vi "Test Animal Cannot Eat after Eating.vi"(8 "error in (no error)":errorcluster, 11 "Animal Test In":refnum<class "Animal Test.lvclass">) -> (0 "error out":errorcluster, 3 "Animal Test Out":refnum<class "Animal Test.lvclass">)   [LabVIEW 2020, in "Animal Test.lvclass"]
doc: "Test Animal cannot eat after eating."
uses:
  Animal Test.lvclass
  C:/Program Files (x86)/National Instruments/LabVIEW 2020/vi.lib/Astemes/LUnit/Test Case.lvclass
  Animal Test.lvclass/Animal Test.ctl
  <vilib>/Astemes/LUnit/Test Case.lvclass/Test Case.ctl
  092653db-4d85-4f60-a039-c6abd7f22ebd.vi
  <vilib>/Astemes/LUnit/Append Fail Result.vi
  <vilib>/Astemes/LUnit/Append Pass Result.vi
  <vilib>/Astemes/LUnit/Compare Variants.vi
  <vilib>/Astemes/LUnit/Describe Comparison.vi
  <vilib>/Astemes/LUnit/Run In UI.vi
  <vilib>/Utility/error.llb/Clear Errors.vi
  <vilib>/Astemes/LUnit/Describe Variant.vi
  Animal Classes/Animal/Animal.lvclass
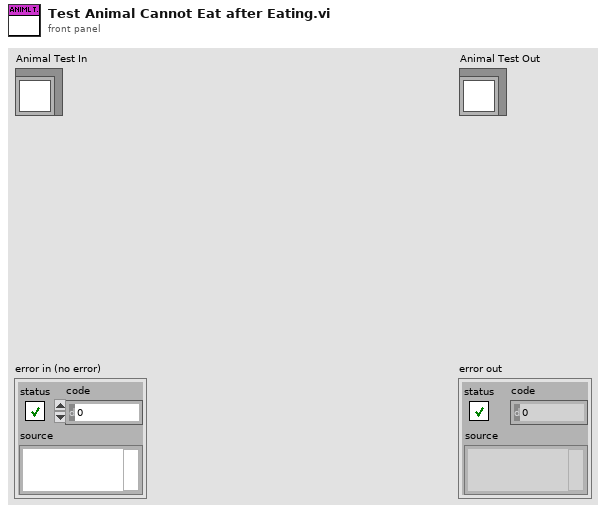
[diagram p1: front panel]
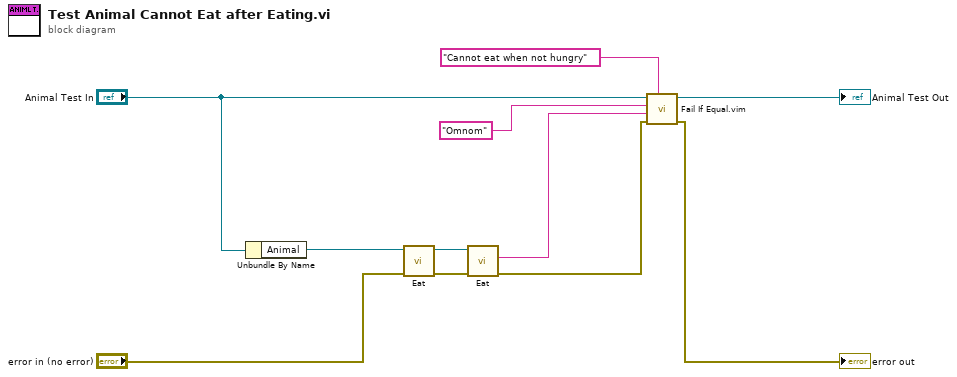
[diagram p0: block diagram]
diagram:
  n1 = Unbundle By Name("Animal Test In") -> ("Animal"=w11:refnum<class "Animal.lvclass">)
  n2 = call-dynamic "Eat.vi"("error in (no error)"="error in (no error)", "Animal In"=w11) -> ("error out"=w9:errorcluster, "Animal Out"=w10:refnum<class "Animal.lvclass">)  [unwired: 7 in, 1 out]
  n3 = call-dynamic "Eat.vi"("error in (no error)"=w9, "Animal In"=w10) -> ("error out"=w2:errorcluster, "Result"=w3:string)  [unwired: 7 in, 1 out]
  n4 = call "Fail If Equal.vim"("Description"="Cannot eat when not hungry", "error in (no error)"=w2, "Actual"=w3, "Unexpected"="Omnom" ("Result"), "LUnit Test Case In"="Animal Test In") -> ("error out"=→"error out":errorcluster, "LUnit Test Case Out"=→"Animal Test Out":refnum<class "Animal Test.lvclass">)  [unwired: 5 in]
